vi "Get State Name.vi"(8 "error in (no error)":errorcluster, 11 "Executing in":refnum<class "Executing.lvclass">) -> (0 "error out":errorcluster, 2 "State Name":string, 3 "Executing out":refnum<class "Executing.lvclass">)   [LabVIEW 2013, in "Command Processor.lvlib" / "Executing.lvclass"]
uses:
  Executing.lvclass
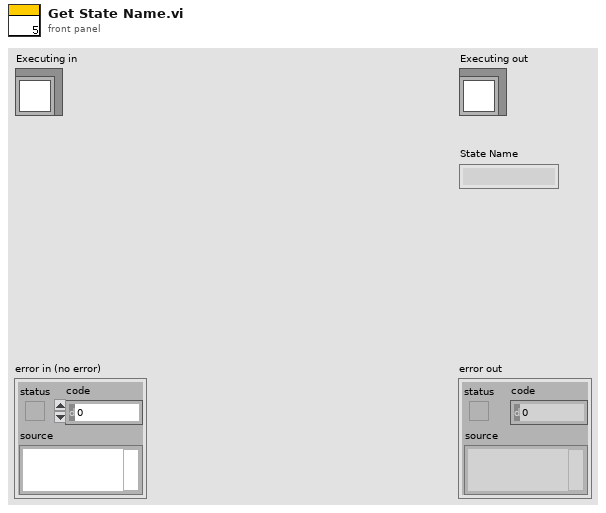
[diagram p1: front panel]
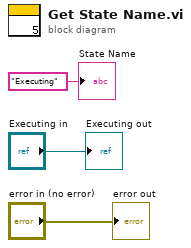
[diagram p0: block diagram]
diagram:
  "error out" <- "error in (no error)"
  "Executing out" <- "Executing in"
  "State Name" <- "Executing" ("State Name")
